vi "PID_LT.vi"() -> ()   [LabVIEW 2019]
uses:
  <vilib>/addons/control/pid/pid.llb/PID Advanced (DBL).vi
  <vilib>/addons/control/pid/NI_PID_pid.lvlib
panel:
  out "Waveform Chart":cluster{"LCV":dbl, "SP":dbl, "Plant Output":dbl}(graph)
  out "LCV":dbl(knob) scale=0.0..100.0
  in  "stop":bool
  in  "process parameters":T1={"static gain"=2.5, "lag (s)"=2.5, "deadtime (s)"=0.001, "load"=0.0, "deadband"=0.0, "sensor noise"=0.0, "initial PV"=30.0, "plant noise"=0.0} {"plant noise" format="%.2f"; "initial PV" format="%.2f"; "sensor noise" format="%.2f"; "lag (s)" format="%.2f"; "deadtime (s)" format="%.2f"; "deadband" format="%.1f"; "load" format="%.2f"; "static gain" format="%.2f"}
  out "PV (Output)":dbl(slide) scale=0.0..100.0
  in  "SP":dbl(slide) scale=0.0..100.0
  in  "PID gains":T2={"proportional gain (Kc)"=1.0, "integral time (Ti, min)"=0.01, "derivative time (Td, min)"=0.0} {"derivative time (Td, min)" format="%.3f"; "integral time (Ti, min)" format="%.3f"; "proportional gain (Kc)" format="%.3f"}
  in  "auto? (T)":bool=TRUE
  in  "LCV":dbl format="%.2f"
  # "LCV"
  # "LT"
  # "Liquid IN"
  # "Liquid OUT"
  # "PID<LT"
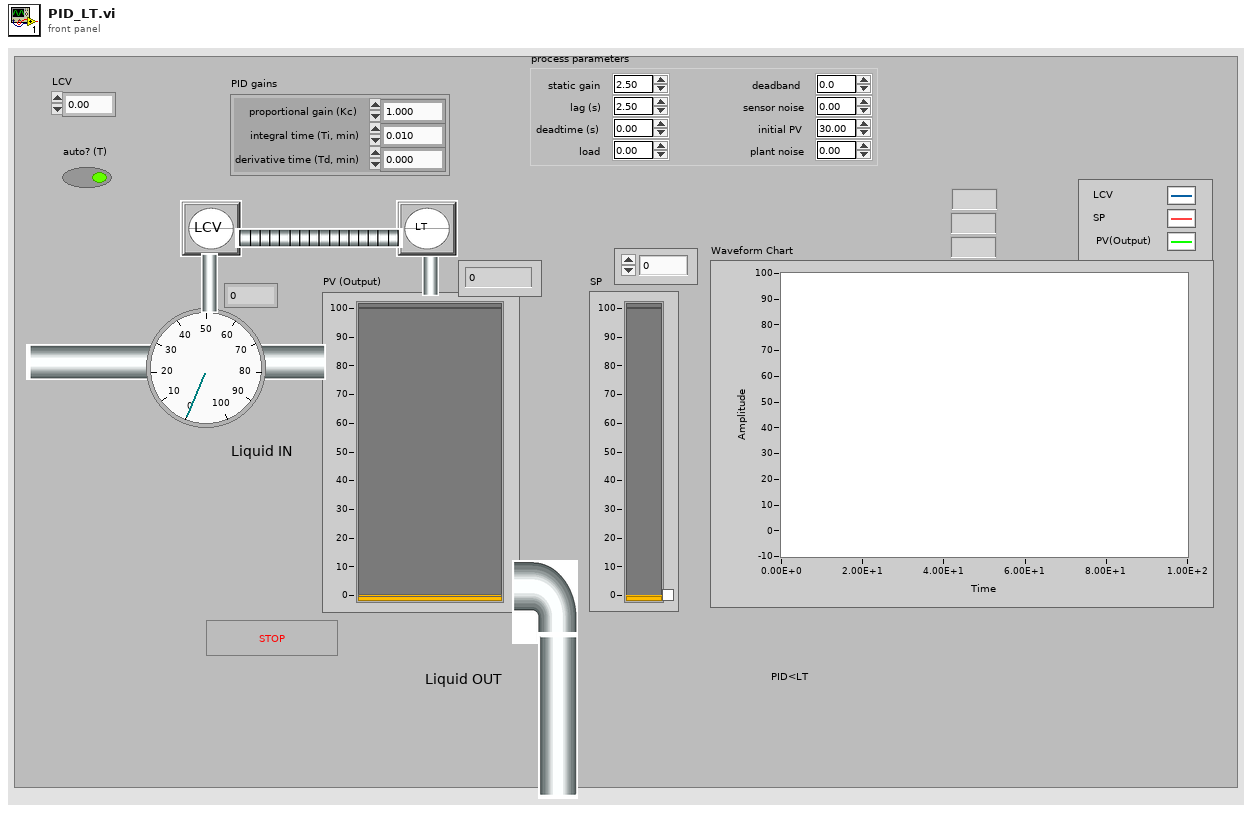
[diagram p1: front panel]
types:
  T1 = cluster{"static gain":dbl, "lag (s)":dbl, "deadtime (s)":dbl, "load":dbl, "deadband":dbl, "sensor noise":dbl, "initial PV":dbl, "plant noise":dbl}
  T2 = cluster{"proportional gain (Kc)":dbl, "integral time (Ti, min)":dbl, "derivative time (Td, min)":dbl}
  T3 = cluster{"output":dbl, "SP":dbl, "Plant Output":dbl}
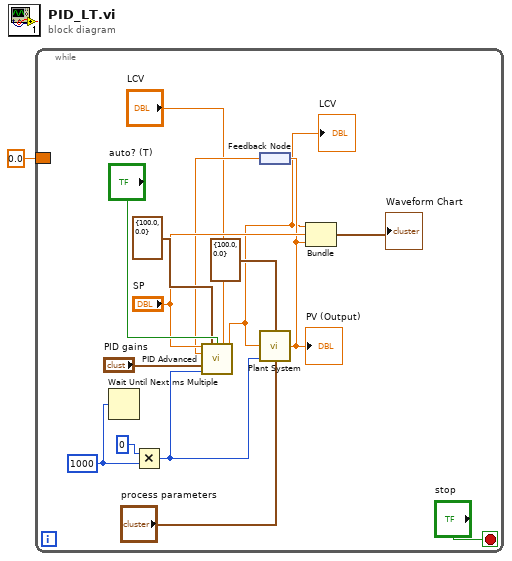
[diagram p0: block diagram]
diagram:
  n1 = while {
    border: 0.0 ("Plant Output") -> [_]
    stop <- "stop" stop-if-true
    w13 = u32 1000 ("millisecond multiple")
    n2 = Wait Until Next ms Multiple(millisecond multiple=w13) -> ()  [unwired: 1 out]
    n3 = Multiply(x=u32 0, y=w13) -> (x*y=w11:u32)
    n4 = feedback #1() -> (w8:dbl)
    n5 = call-poly <vilib>:"PID Advanced.vi"("setpoint"="SP", "output range"=cluster{"output high":dbl, "output low":dbl} {"output high"=100.0, "output low"=0.0}, "auto? (T)"="auto? (T)", "manual control"="LCV", "process variable"=w8, "PID gains"="PID gains", "dt (s)"=w11) -> ("output"=w2:dbl)  [unwired: 7 in, 1 out]
    "LCV" <- w2
    n6 = call "Plant System.vi"("output saturation range"=cluster{"output high":dbl, "output low":dbl} {"output high"=100.0, "output low"=0.0}, "Plant Input"=w2, "dt (s)"=w11, "process parameters"="process parameters") -> ("Plant Output"=w7:dbl)  [unwired: 11 in]
    "PV (Output)" <- w7
    n7 = feedback-in #1(w7) -> ()
    n8 = Bundle("output"=w2, "SP"="SP", "Plant Output"=w7) -> (→"Waveform Chart":T3)  [unwired: 1 in]
  }
